vi "Untitled 1.vi"() -> ()   [LabVIEW 2023]
panel:
  out "Gauge":dbl(knob) scale=0.0..2000.0
  out "Thermometer":dbl(slide) scale=0.0..100.0
  out "Tank":dbl(slide) scale=0.0..1000.0
  out "Time Stamp 2":timestamp
  in  "Time Stamp":timestamp
  out "Numeric 2":dbl
  in  "Numeric":dbl
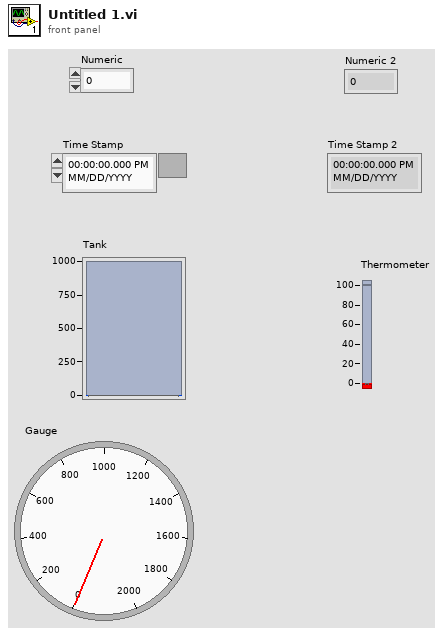
[diagram p1: front panel]
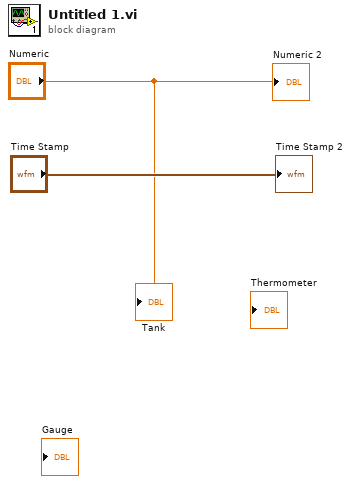
[diagram p0: block diagram]
diagram:
  "Numeric 2" <- "Numeric"
  "Time Stamp 2" <- "Time Stamp"
  "Tank" <- "Numeric"
